vi "Cal Freq.vi"(7 "sample":u32, 8 "error in (no error)":errorcluster, 9 "voltage_resolution":dbl, 10 "buffer_length":u32, 11 "buffer":dbl) -> (0 "error out":errorcluster, 2 "function return":i32, 3 "buffer out":dbl)   [LabVIEW 2021, in "vmmso.lvlib"]
doc: "DLL_API int WINAPI CalFreq(double* buffer, unsigned int buffer_length, double voltage_resolution, unsigned int sample);"
uses:
  vmmso.lvlib
  vmmso.dll
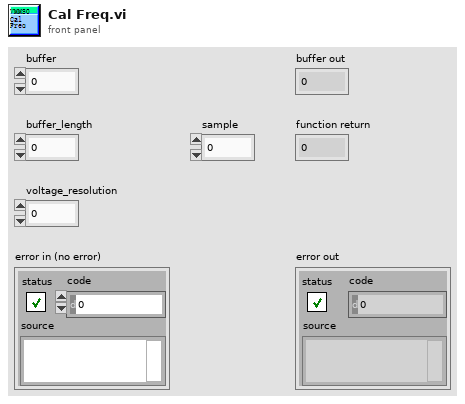
[diagram p1: front panel]
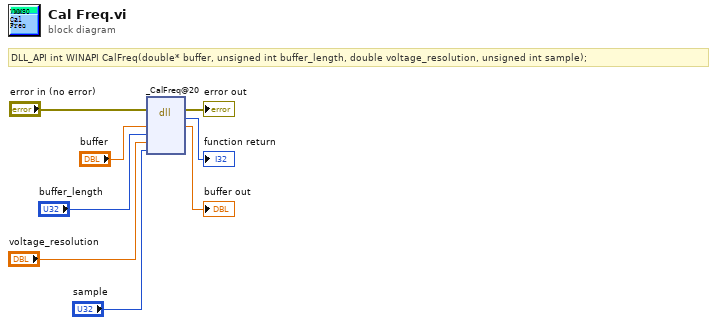
[diagram p0: block diagram]
diagram:
  # "DLL_API int WINAPI CalFreq(double* buffer, unsigned int buffer_length, double voltage_resolution, unsigned int sample);"
  n1 = dll-call lib="O:/MSO/library/demo-Labview/vmmso/vmmso.*" fn="_CalFreq@20"(error in="error in (no error)", "buffer"="buffer", "buffer_length"="buffer_length", "voltage_resolution"="voltage_resolution", "sample"="sample") -> (error out=→"error out":errorcluster, →"function return":i32, "buffer"=→"buffer out":dbl)  [unwired: 5 in, 1 out]
